vi "Get Application Instance Details.vi"(5 "Application Instance Ref":refnum<vi>) -> (0 "This Application Reference":u32, 1 "VI Of Top-Most Block Diagram":string, 2 "Application Name":string)   [LabVIEW 2022 SP3]
doc: "<add documentation here>"
panel:
  # "Development\nControls or indicators that are useful for development or testing, but which are not outputs of the VI."
  # "Input\nInputs to the VI"
  # "Output\nOutputs of the VI"
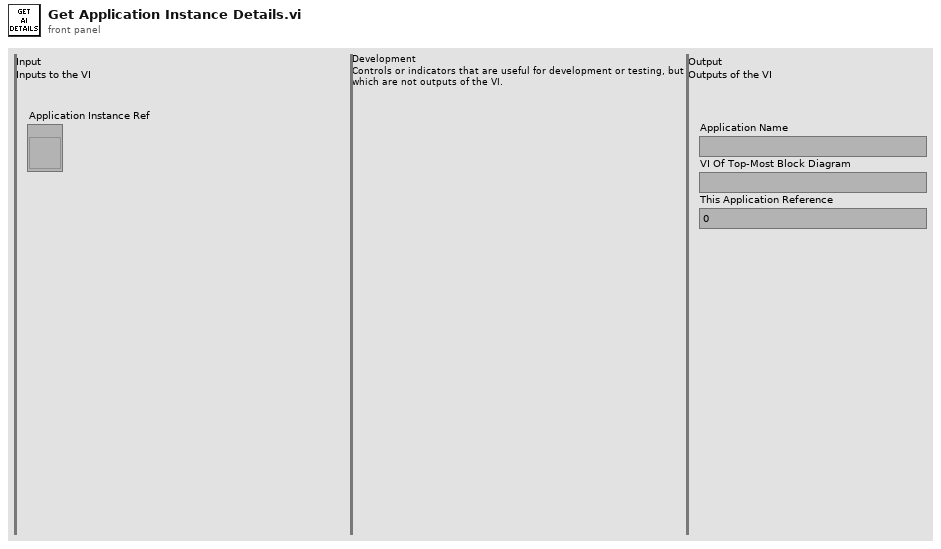
[diagram p1: front panel]
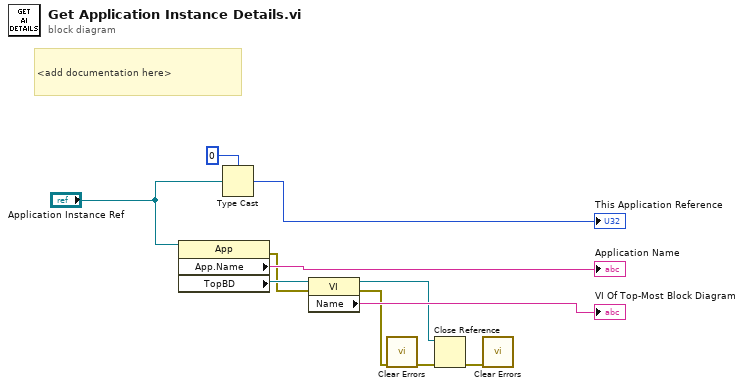
[diagram p0: block diagram]
diagram:
  # "<add documentation here>"
  n1 = property class="App"(reference="Application Instance Ref") -> (error out=w6:errorcluster, "App.Name"=→"Application Name":string, "TopBD"=w11:refnum<vi>)  [unwired: 1 in, 1 out]
  n2 = Type Cast(type=u32 0, x="Application Instance Ref") -> (*(type *) &x=→"This Application Reference":u32)
  n3 = property class="VI"(reference=w11, error in=w6) -> (reference out=w3:refnum<vi>, error out=w5:errorcluster, "Name"=→"VI Of Top-Most Block Diagram":string)
  n4 = call <vilib>:"Clear Errors.vi"("error in (no error)"=w5) -> ("error out"=w4:errorcluster)  [unwired: 5 in, 1 out]
  n5 = Close Reference(reference=w3, error in (no error)=w4) -> (error out=w1:errorcluster)
  n6 = call <vilib>:"Clear Errors.vi"("error in (no error)"=w1) -> ()  [unwired: 5 in, 2 out]
